vi "oax_Reset Selected Devices.vi"(8 "error in":errorcluster, 11 "devices to reset":string[](array[string])) -> (0 "error out":errorcluster)   [LabVIEW 2017]
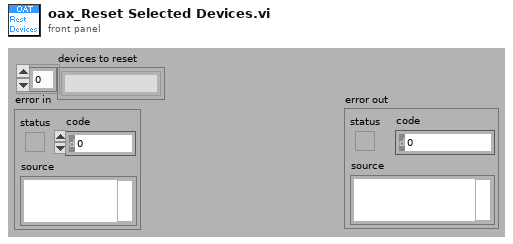
[diagram p1: front panel]
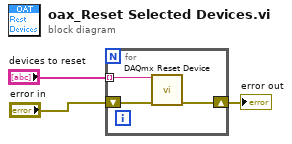
[diagram p0: block diagram]
diagram:
  n1 = for {
    tunnel: "devices to reset" -> [w6] mode=indexing
    shift-right: [w4] -> w1
    shift-left: "error in" -> [w5]
    n2 = call <vilib>:"DAQmx Reset Device.vi"("device in"=w6, "error in"=w5) -> ("error out"=w4:errorcluster)  [unwired: 13 in]
  }
  "error out" <- w1
